vi "Prepare Monkeys from Jobs.vi"(0 "Monkey Jobs":string[](array[string]), 1 "Bored Operation":string="/ 3") -> (3 "Monkeys":T1)   [LabVIEW 2020, in "AoC 2022.lvlib"]
uses:
  AoC 2022.lvlib
  Day 11 - Monkey in the Middle/private/Monkeys.ctl
  Day 11 - Monkey in the Middle/private/Monkey.ctl
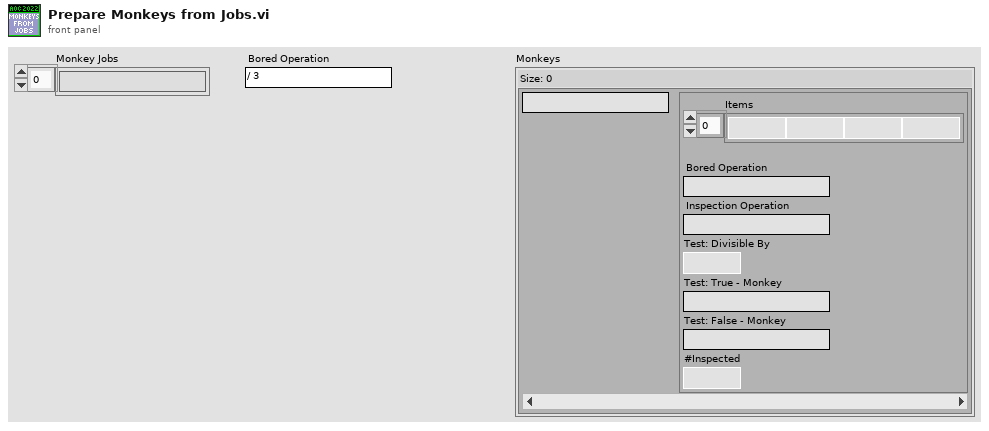
[diagram p1: front panel]
types:
  T1 = typedef "AoC 2022.lvlib/Monkeys.ctl" = map{string, T2}
  T2 = typedef "AoC 2022.lvlib/Monkey.ctl" = cluster{"Items":u64[], "Bored Operation":string, "Inspection Operation":string, "Test: Divisible By":u64, "Test: True - Monkey":string, "Test: False - Monkey":string, "#Inspected":i32}
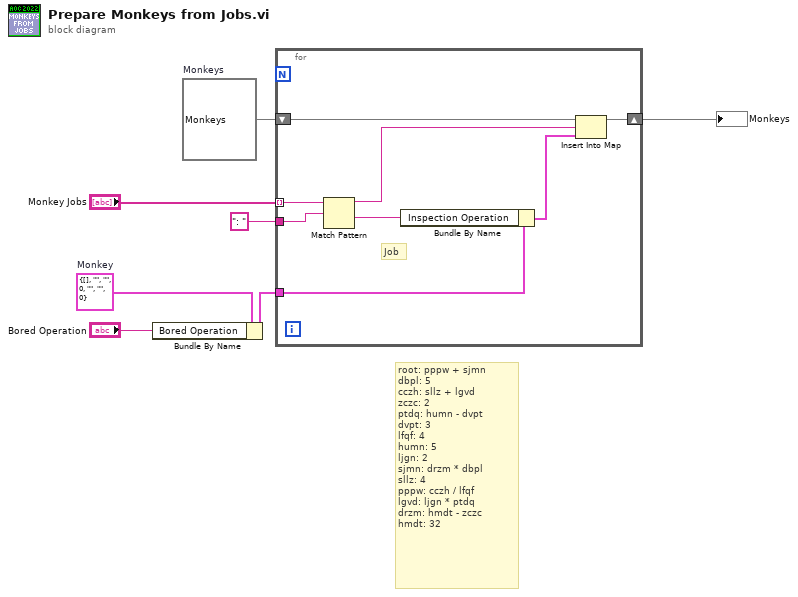
[diagram p0: block diagram]
diagram:
  w6 = T2 {"Items"=[], "Bored Operation"="", "Inspection Operation"="", "Test: Divisible By"=0, "Test: True - Monkey"="", "Test: False - Monkey"="", "#Inspected"=0}  # Monkey
  w5 = T1 {}  # Monkeys
  # "root: pppw + sjmn\ndbpl: 5\ncczh: sllz + lgvd\nzczc: 2\nptdq: humn - dvpt\ndvpt: 3\nlfqf: 4\nhumn: 5\nljgn: 2\nsjmn: drzm * dbpl\nsllz: 4\npppw: cczh / lfqf\nlgvd: ljgn * ptdq\ndrzm: hmdt - zczc\nhmdt: 32"
  n1 = Bundle By Name(cluster=w6, "Bored Operation"="Bored Operation") -> (w3:T2)
  n2 = for {
    shift-right: [w14] -> w1
    shift-left: w5 -> [w15]
    tunnel: w3 -> [w13]
    tunnel: ": " -> [w10]
    tunnel: "Monkey Jobs" -> [w11] mode=indexing
    # "Job"
    n3 = Match Pattern(string=w11, regular expression=w10) -> (before substring=w9:string, after substring=w8:string)  [unwired: 1 in, 2 out]
    n4 = Bundle By Name(cluster=w13, "Inspection Operation"=w8) -> (w12:T2)
    n5 = Insert Into Map(map in=w15, key=w9, value=w12) -> (map out=w14:T1)  [unwired: 2 out]
  }
  "Monkeys" <- w1
